vi "Conversione di numeri in diverse basi.vi"() -> ()   [LabVIEW 2013]
panel:
  in  "stop":bool
  out "Array 2":dbl[](array[numeric])
  out "Array":dbl[](array[numeric])
  in  "base convertitore":dbl
  in  "base 10":dbl
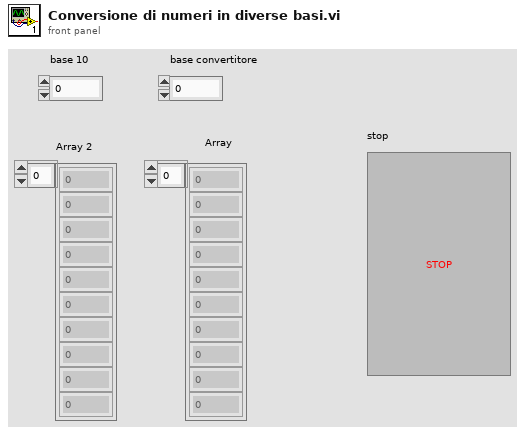
[diagram p1: front panel]
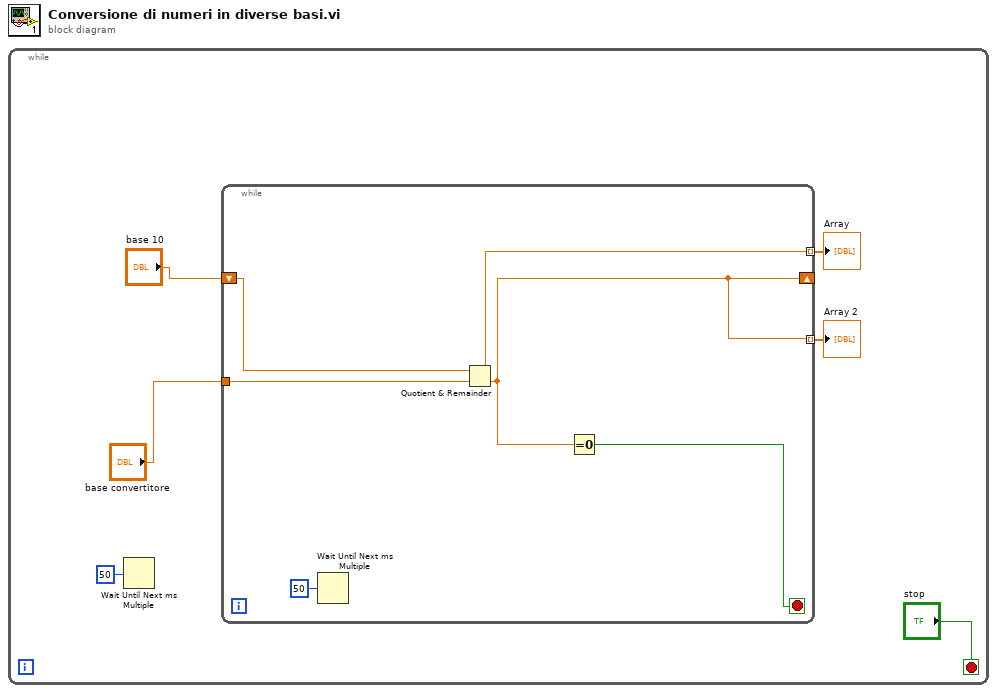
[diagram p0: block diagram]
diagram:
  n1 = while {
    stop <- "stop" stop-if-true
    n2 = Wait Until Next ms Multiple(millisecond multiple=u32 50 ("millisecond timer value")) -> ()  [unwired: 1 out]
    n3 = while {
      shift-right: [w8] -> _
      shift-left: "base 10" -> [w10]
      tunnel: "base convertitore" -> [w11]
      tunnel: [w9] -> w4 mode=indexing
      tunnel: [w8] -> w3 mode=indexing
      stop <- w7 stop-if-true
      n4 = Wait Until Next ms Multiple(millisecond multiple=u32 50) -> ()  [unwired: 1 out]
      n5 = Quotient & Remainder(x=w10, y=w11) -> (x-y*floor(x/y)=w9:dbl, floor(x/y)=w8:dbl)
      n6 = Equal To 0?(x=w8) -> (x = 0?=w7:bool)
    }
    "Array" <- w4
    "Array 2" <- w3
  }
